vi "Transform.vi"(7 "Type X":T2(ring), 8 "error in (no error)":errorcluster caption="entrée d'erreur (pas d'erreur)", 9 "y":string[][](array[string]), 10 "X":string[][](array[string]), 11 "TfidfTransformer.lvclass":refnum<class "TfidfTransformer.lvclass">) -> (0 "error out":errorcluster caption="sortie d'erreur", 2 "Data":T1, 3 "TfidfTransformer.lvclass":refnum<class "TfidfTransformer.lvclass">)   [LabVIEW 2020, in "TfidfTransformer.lvclass"]
doc: "Transform a count matrix to a tf or tf-idf representation\n\nReturns : \n\n- vectors : sparse matrix of shape (n_samples, n_features)"
uses:
  TfidfTransformer.lvclass
  TfidfTransformer.lvclass/TfidfTransformer.ctl
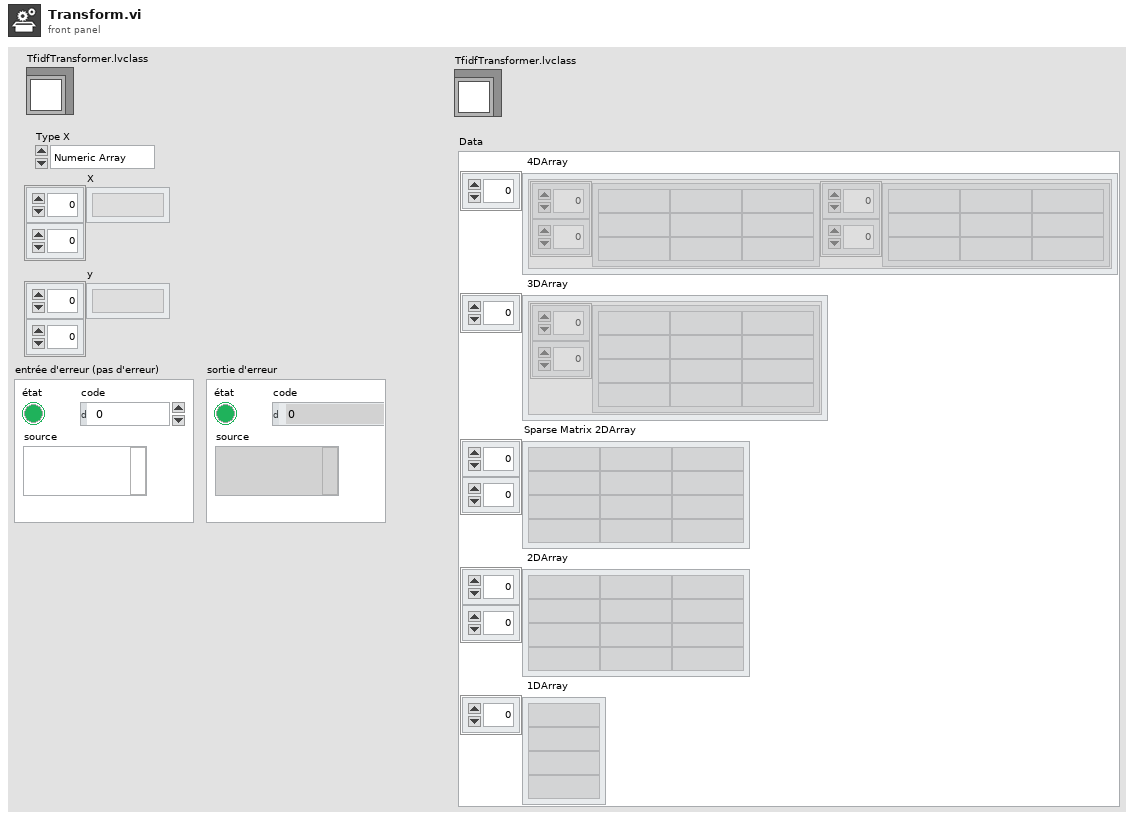
[diagram p1: front panel]
types:
  T1 = cluster{" 4DArray":cluster{"1":string[][], "2":string[][]}[], " 3DArray":cluster{"Tableau":string[][]}[], "Sparse Matrix 2DArray":string[][], " 2DArray":string[][], " 1DArray":string[]}
  T2 = enum16{"Numeric Array", "String Array", "Sparse"}
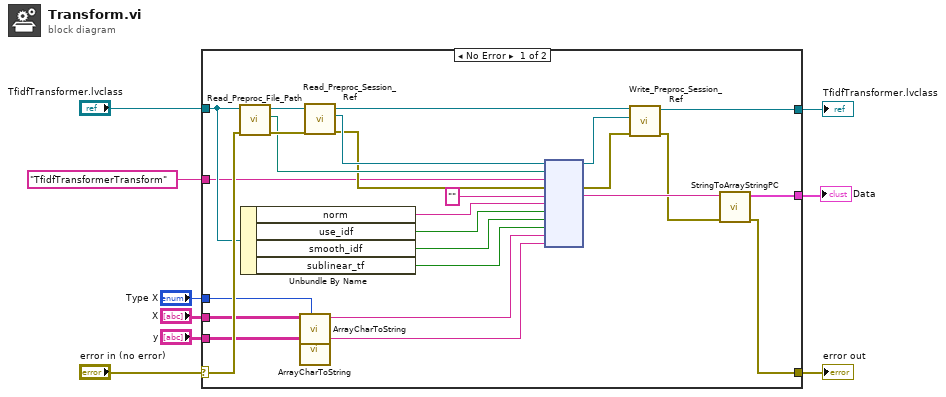
[diagram p0: block diagram]
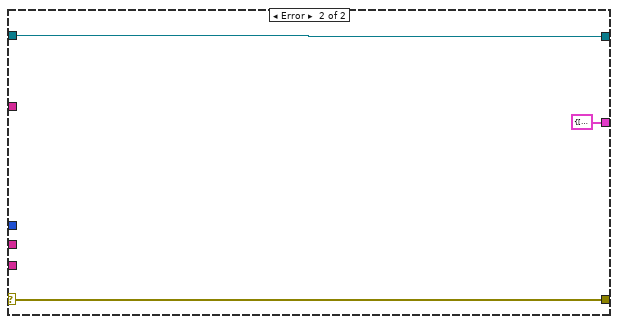
[diagram p2: hidden frame]
diagram:
  n1 = case shown="No Error" "error in (no error)" {
    selector: "error in (no error)" -> [w26 w38]
    tunnel: [w10 w38] -> w8
    tunnel: [w13 w37] -> w6
    tunnel: "TfidfTransformer.lvclass" -> [w25 w37]
    tunnel: "TfidfTransformerTransform" ("Fonction") -> [w24 _]
    tunnel: [w11 T1 {" 4DArray"=[], " 3DArray"=[], "Sparse Matrix 2DArray"=[], " 2DArray"=[], " 1DArray"=[]} ("Data")] -> w1
    tunnel: "X" -> [w19 _]
    tunnel: "y" -> [w18 _]
    tunnel: "Type X" -> [w15 _]
    frame No Error {
      n2 = call-dynamic "Read_Preproc_File_Path.vi"("error in (no error)"=w26, "Python in"=w25) -> ("error out"=w34:errorcluster, "File_Path"=w33:path, "Python out"=w35:refnum<class "TfidfTransformer.lvclass">)  [unwired: 7 in]
      n3 = Unbundle By Name(w25) -> ("norm"=w23:string, "use_idf"=w22:bool, "smooth_idf"=w21:bool, "sublinear_tf"=w20:bool)
      n4 = call "ArrayCharToString.vi"("Type"=w15, "TAB"=w19) -> ("Instruction"=w17:string)  [unwired: 9 in]
      n5 = call "ArrayCharToString.vi"("TAB"=w18) -> ("Instruction"=w16:string)  [unwired: 10 in]
      n6 = call-dynamic "Read_Preproc_Session_Ref.vi"("error in (no error)"=w34, "Python in"=w35) -> ("error out"=w31:errorcluster, "Session_ref"=w32:refnum<k35>, "Python out"=w30:refnum<class "TfidfTransformer.lvclass">)  [unwired: 7 in]
      n7 = node(w32, w33, w24, w31, "", w23, w22, w21, w20, w17, w16) -> (w28:refnum<k35>, w29:errorcluster, w14:string)  [unwired: 6 in, 2 out]
      n8 = call-dynamic "Write_Preproc_Session_Ref.vi"("error in (no error)"=w29, "Session_ref"=w28, "Python in"=w30) -> ("error out"=w12:errorcluster, "Python out"=w13:refnum<class "TfidfTransformer.lvclass">)  [unwired: 7 in]
      n9 = call "StringToArrayStringPC.vi"("sortie d'erreur"=w12, "Return value"=w14) -> ("sortie d'erreur"=w10:errorcluster, "Data"=w11:T1)  [unwired: 8 in]
    }
    frame Error {
    }
  }
  "error out" <- w8
  "TfidfTransformer.lvclass" <- w6
  "Data" <- w1
